vi "Write Address Recursive Access.vi"(8 "error in (no error)":errorcluster, 10 "Address":i32[](array[numeric]), 11 "Simple Tree Queue Mailman in":refnum<class "Simple Tree Queue Mailman.lvclass">) -> (0 "error out":errorcluster, 3 "Simple Tree Queue Mailman out":refnum<class "Simple Tree Queue Mailman.lvclass">)   [LabVIEW 2024, in "Simple Tree Queue Mailman.lvclass"]
uses:
  Simple Tree Queue Mailman.lvclass
  Simple Tree Queue Mailman.lvclass/Simple Tree Queue Mailman.ctl
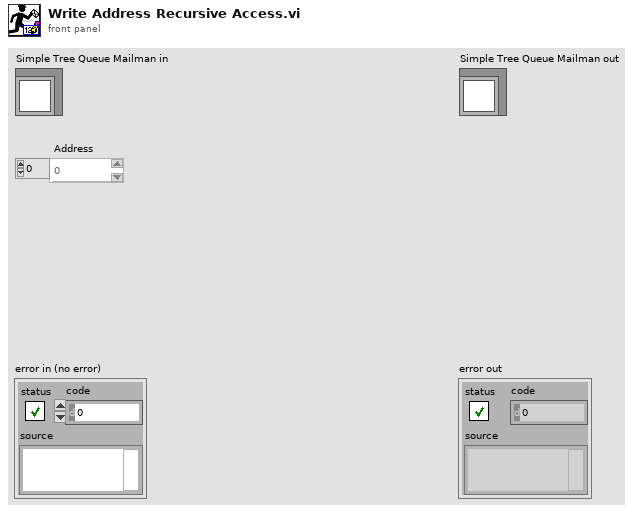
[diagram p1: front panel]
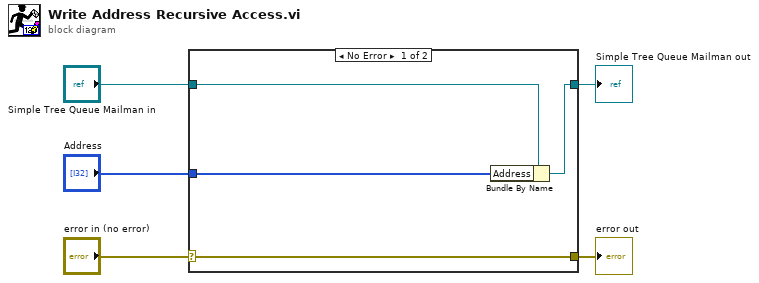
[diagram p0: block diagram]
diagram:
  n1 = case shown="No Error" "error in (no error)" {
    selector: "error in (no error)" -> [w9 w10]
    tunnel: [w9 w10] -> w4
    tunnel: [w7 w11] -> w2
    tunnel: "Simple Tree Queue Mailman in" -> [w8 w11]
    tunnel: "Address" -> [w6 _]
    frame No Error {
      n2 = Bundle By Name(cluster=w8, "Address"=w6) -> (w7:refnum<class "Simple Tree Queue Mailman.lvclass">)
    }
    frame Error {
    }
  }
  "error out" <- w4
  "Simple Tree Queue Mailman out" <- w2
